vi "load_single_image.vi"(8 "error in (no error)":errorcluster, 11 "data_loder_single_image in":refnum<class "data_loder_single_image.lvclass">) -> (0 "error out":errorcluster, 3 "data_loder_single_image out":refnum<class "data_loder_single_image.lvclass">)   [LabVIEW 2017, in "data_loder_single_image.lvclass"]
uses:
  data_loder_single_image.lvclass
  data_loder_single_image.lvclass/data_loder_single_image.ctl
panel:
  out "secondary list":string[](array[string])
  out "record the secondary name":bool
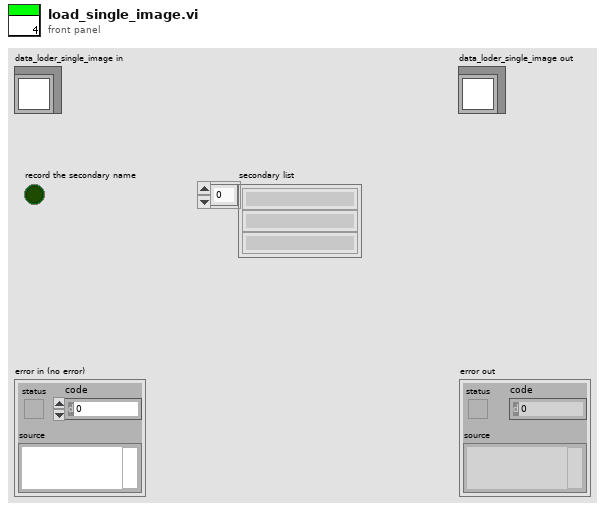
[diagram p1: front panel]
types:
  T1 = typedef "imagedata.ctl" = cluster{"image type":i32, "image depth":i32, "image":u8[], "mask":u8[], "colors":u32[], "Rectangle":cluster{"left":i16, "top":i16, "right":i16, "bottom":i16}}
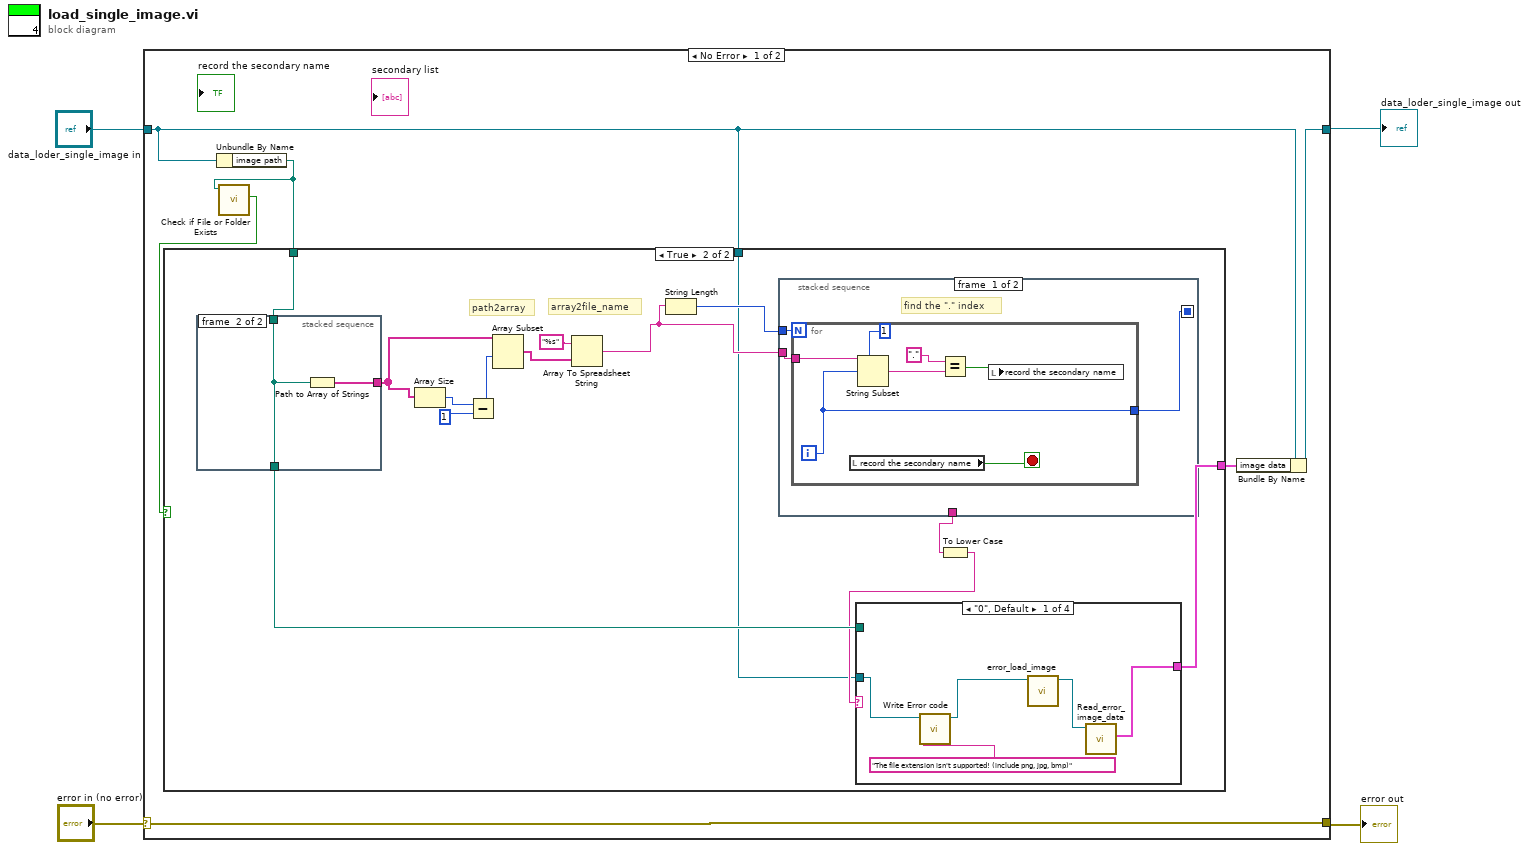
[diagram p0: block diagram]
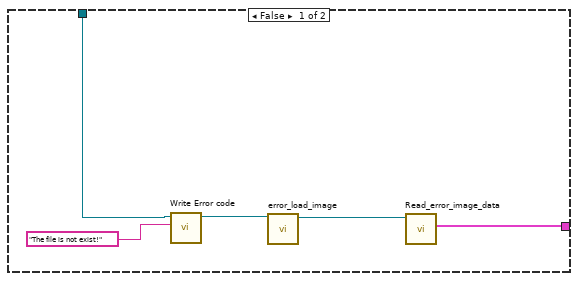
[diagram p2: hidden frame]
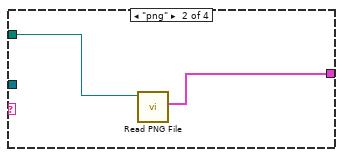
[diagram p3: hidden frame]
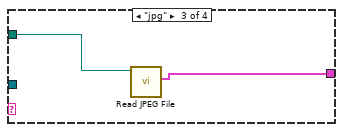
[diagram p4: hidden frame]
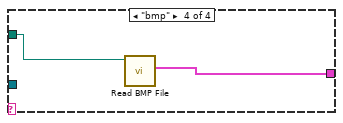
[diagram p5: hidden frame]
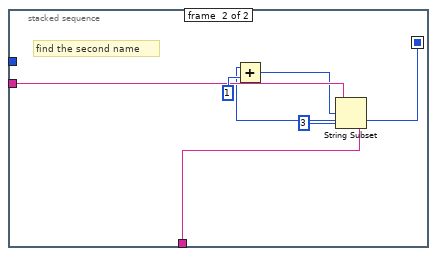
[diagram p6: hidden frame]
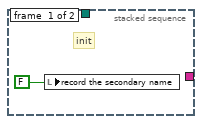
[diagram p7: hidden frame]
diagram:
  n1 = case shown="No Error" "error in (no error)" {
    selector: "error in (no error)" -> [w10 w61]
    tunnel: [w10 w61] -> w3
    tunnel: [w8 w60] -> w1
    tunnel: "data_loder_single_image in" -> [w7 w60]
    frame No Error {
      n2 = Unbundle By Name(w7) -> ("image path"=w6:path)
      n3 = call <vilib>:"Check if File or Folder Exists.vi"("path"=w6) -> ("file or folder exists?"=w5:bool)  [unwired: 8 in, 2 out]
      n4 = case shown="True" w5 {
        tunnel: [w14 w18] -> w9
        tunnel: w7 -> [w12 w17]
        tunnel: w6 -> [_ w16]
        frame False {
          n5 = call-dynamic "Write Error code.vi"("Error code"="The file is not exist!", "data_loader in"=w12) -> ("data_loader out"=w11:refnum<class "data_loder_single_image.lvclass">)  [unwired: 8 in, 1 out]
          n6 = call-dynamic "error_load_image.vi"("data_loader in"=w11) -> ("data_loader out"=w15:refnum<class "data_loder_single_image.lvclass">)  [unwired: 9 in, 1 out]
          n7 = call-dynamic "Read_error_image_data.vi"("data_loader in"=w15) -> ("image data"=w14:T1)  [unwired: 8 in, 2 out]
        }
        frame True {
          # "array2file_name"
          # "path2array"
          n8 = stacked-sequence {
            tunnel: w16 -> [_ w58]
            tunnel: [_ w59] -> w19
            tunnel: [_ w58] -> w22
            frame #0 {
              # "init"
              n9 = local write "record the secondary name"(FALSE) -> ()
            }
            frame #1 {
              n10 = Path to Array of Strings(0:w58) -> (2:w59:string[])  [unwired: 1 out]
            }
          }
          n11 = Array Size(array=w19) -> (size(s)=w28:i32)
          n12 = Subtract(x=w28, y=1) -> (x-y=w27:i32)
          n13 = Array Subset(array=w19, index=w27) -> (w26:string[])  [unwired: 1 in]
          n14 = Array To Spreadsheet String(array=w26, 3:"%s" ("format string")) -> (spreadsheet string=w24:string)  [unwired: 1 in]
          n15 = String Length(string=w24) -> (length=w23:i32)
          n16 = stacked-sequence {
            seq-local: [w41 _] -> [_ w52]
            tunnel: w24 -> [w43 w54]
            tunnel: w23 -> [w42 _]
            tunnel: [_ w55] -> w21
            frame #0 {
              # "find the \".\" index"
              n17 = for {
                N: w42 -> [_]
                tunnel: w43 -> [w50]
                tunnel: [w44] -> w41
                i -> [w44]
                stop <- w45 stop-if-true
                n18 = local read "record the secondary name"() -> (w45:bool)
                n19 = String Subset(string=w50, offset (0)=w44, length (rest)=1 ("length (rest)")) -> (substring=w46:string)
                n20 = Equal?(x=".", y=w46) -> (x = y?=w47:bool)
                n21 = local write "record the secondary name"(w47) -> ()
              }
            }
            frame #1 {
              # "find the second name"
              n22 = Add(x=w52, y=1) -> (x+y=w53:i32)
              n23 = String Subset(string=w54, offset (0)=w53, length (rest)=3) -> (substring=w55:string)
            }
          }
          n24 = To Lower Case(string=w21) -> (all lower case string=w20:string)
          n25 = case shown="\"0\", Default" w20 {
            tunnel: w22 -> [_ w36 w38 w39]
            tunnel: [w33 w35 w37 w40] -> w18
            tunnel: w17 -> [w31 _ _ _]
            frame "0", Default {
              n26 = call-dynamic "Write Error code.vi"("Error code"="The file extension isn't supported! (include png, jpg, bmp)", "data_loader in"=w31) -> ("data_loader out"=w30:refnum<class "data_loder_single_image.lvclass">)  [unwired: 8 in, 1 out]
              n27 = call-dynamic "error_load_image.vi"("data_loader in"=w30) -> ("data_loader out"=w34:refnum<class "data_loder_single_image.lvclass">)  [unwired: 9 in, 1 out]
              n28 = call-dynamic "Read_error_image_data.vi"("data_loader in"=w34) -> ("image data"=w33:T1)  [unwired: 8 in, 2 out]
            }
            frame "png" {
              n29 = call <vilib>:"Read PNG File.vi"("path to PNG file"=w36) -> ("image data"=w35:T1)  [unwired: 8 in, 2 out]
            }
            frame "jpg" {
              n30 = call <vilib>:"Read JPEG File.vi"("path to JPEG file"=w38) -> ("image data"=w37:T1)  [unwired: 8 in, 2 out]
            }
            frame "bmp" {
              n31 = call <vilib>:"Read BMP File.vi"("path to BMP file"=w39) -> ("image data"=w40:T1)  [unwired: 8 in, 2 out]
            }
          }
        }
      }
      n32 = Bundle By Name(cluster=w7, "image data"=w9) -> (w8:refnum<class "data_loder_single_image.lvclass">)
    }
    frame Error {
    }
  }
  "error out" <- w3
  "data_loder_single_image out" <- w1
